vi "Save Reference Rectangle.vi"(8 "error in (no error)":errorcluster, 11 "Z-Plane":i32 format="Plane %.0f") -> (0 "error out":errorcluster)   [LabVIEW 2017]
uses:
  <vilib>/Utility/error.llb/whitespace.ctl
  Globals/gl_Movement correction globals.vi
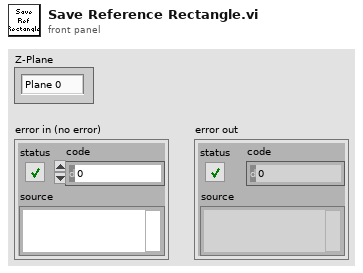
[diagram p1: front panel]
types:
  T1 = typedef "Reference_Globals.ctl" = cluster{"Refrence data path":path, "Reference Rectangle":i16[][], "AOL Z":dbl, "No of pixels in a miniscan ":i32[], "Threshold":i16[], "No of miniscans":i32[], "Full Frame Size":u16, "Reference Image":T2, "dwelltime":dbl, "Zoom":dbl, "Field of View":dbl}
  T2 = typedef "IMAQ Image.ctl" = refnum<image>
  T3 = typedef "whitespace.ctl" = u16
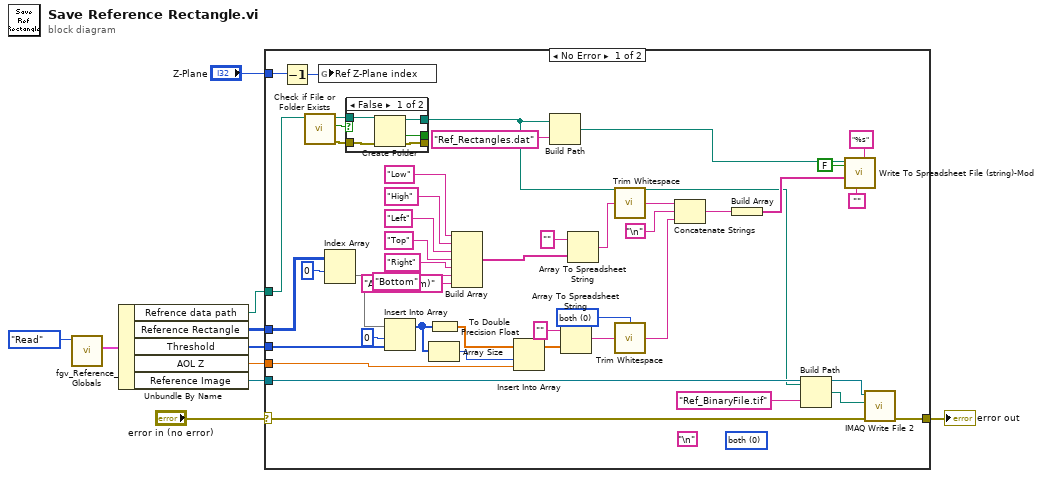
[diagram p0: block diagram]
diagram:
  n1 = call "fgv_Reference_Globals.vi"("Function"=enum16{"Intialize", "Write", "Read", "Clear"}."Read") -> ("Reference Data"=w7:T1)  [unwired: 9 in, 1 out]
  n2 = Unbundle By Name(w7) -> ("Refrence data path"=w6:path, "Reference Rectangle"=w5:i16[][], "Threshold"=w4:i16[], "AOL Z"=w3:dbl, "Reference Image"=w2:T2)
  n3 = case shown="No Error" "error in (no error)" {
    selector: "error in (no error)" -> [w52 w62]
    tunnel: [w51 w62] -> w9
    tunnel: w6 -> [w15 _]
    tunnel: w5 -> [w44 _]
    tunnel: w3 -> [w23 _]
    tunnel: w4 -> [w26 _]
    tunnel: w2 -> [w25 _]
    tunnel: "Z-Plane" -> [w12 _]
    frame No Error {
      (unwired) T3 0 items=["both", "start of string", "end of string"] ("location (both)")
      (unwired) "\n"
      w47 = T3 0 items=["both", "start of string", "end of string"] ("location (both)")
      n4 = Decrement(x=w12) -> (x-1=w11:i32)
      n5 = call <vilib>:"Check if File or Folder Exists.vi"("path"=w15) -> ("error out"=w17:errorcluster, "file or folder exists?"=w18:bool, "dup path"=w16:path)  [unwired: 8 in]
      n6 = global write "gl_Movement correction globals.vi" "Ref Z-Plane index"(w11) -> ()
      n7 = Index Array(array=w44, index (row)=0) -> (element=w43:i16[])  [unwired: 1 in]
      n8 = case shown="False" w18 {
        tunnel: w16 -> [w60 w61]
        tunnel: w17 -> [w59 _]
        tunnel: [w58 w61] -> w14
        tunnel: [w57 _] -> _
        tunnel: [w56 _] -> _
        frame False {
          n9 = Create Folder(path (use dialog)=w60, error in=w59) -> (created path=w58:path, cancelled=w56:bool, error out=w57:errorcluster)  [unwired: 1 in]
        }
        frame True {
        }
      }
      n10 = Insert Into Array "Insert Into Array"(array=w43, index=0 ("disabled index (col)"), new element=w26) -> (w21:i16[])
      n11 = Array Size(array=w21) -> (size(s)=w20:i32)
      n12 = To Double Precision Float(number=w21) -> (double precision float=w22:dbl[])
      n13 = Build Array("Low" ("string"), "High" ("string"), "Left" ("string"), "Top" ("string"), "Right" ("string"), "Bottom" ("string"), "AOL Z (norm)" ("element")) -> (w40:string[])
      n14 = Insert Into Array(array=w22, index=w20, new element=w23) -> (w24:dbl[])
      n15 = Build Path(base path=w14, name or relative path="Ref_Rectangles.dat") -> (appended path=w55:path)
      n16 = Array To Spreadsheet String(array=w24, 3:"" ("format string")) -> (spreadsheet string=w50:string)  [unwired: 1 in]
      n17 = Array To Spreadsheet String(array=w40, 3:"" ("format string")) -> (spreadsheet string=w31:string)  [unwired: 1 in]
      n18 = call <vilib>:"Trim Whitespace.vi"("string"=w31) -> ("trimmed string"=w30:string)  [unwired: 1 in]
      n19 = call <vilib>:"Trim Whitespace.vi"("string"=w50, "location (both)"=w47) -> ("trimmed string"=w48:string)
      n20 = Concatenate Strings(w30, "\n", w48) -> (w28:string)
      n21 = Build Array(w28) -> (w27:string[])
      n22 = Build Path(base path=w14, name or relative path="Ref_BinaryFile.tif") -> (appended path=w53:path)
      n23 = call <userlib>:"Write To Spreadsheet File (string)-Mod.vi"("format (%s)"="%s", "delimiter (\\t)"="" ("delimiter (\\t)"), "append to file? (new file:F)"=FALSE, "1D data"=w27, "file path (dialog if empty)"=w55) -> ()  [unwired: 5 in, 2 out]
      n24 = call-poly "IMAQ Write File 2"("error in (no error)"=w52, "File Path"=w53, "Image"=w25) -> ("error out"=w51:errorcluster)  [unwired: 7 in, 1 out]
    }
    frame Error {
    }
  }
  "error out" <- w9
